vi "grain bin indicator debug.vi"() -> ()   [LabVIEW 2020]
panel:
  out "Numeric 2":dbl caption="bu"
  out "Numeric":dbl caption="bu"
  out "Boolean":bool
  out "Boolean 2":bool
  out "Boolean 4":bool
  out "Boolean 3":bool
  out "Slide 3":cluster{u8, u8}(slide)={0, 61}
  # "Dry Bin Storage"
  # "Dryer Bin"
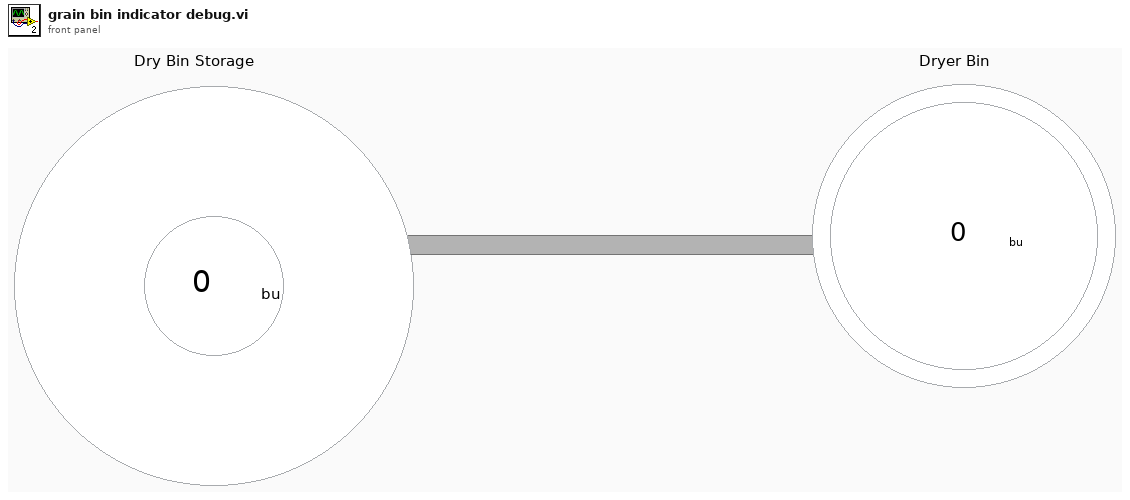
[diagram p1: front panel]
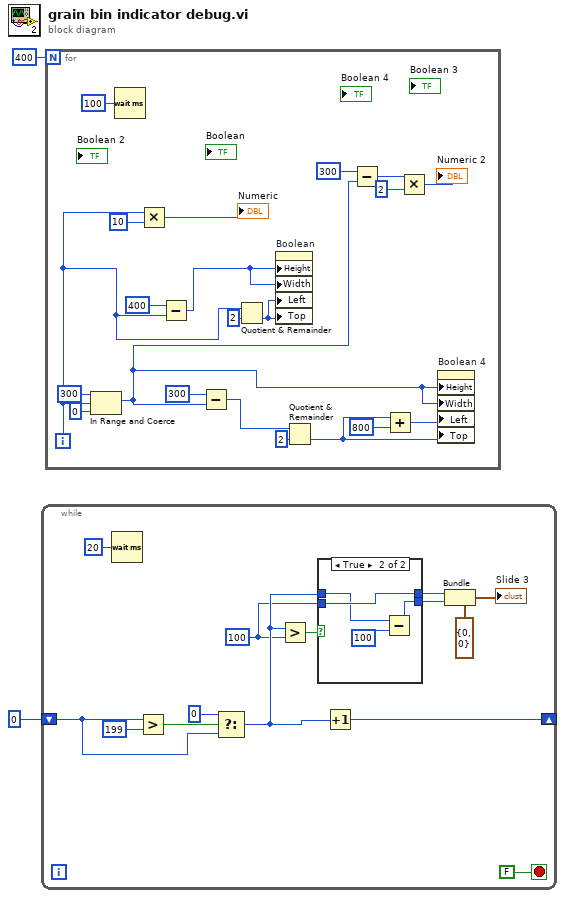
[diagram p0: block diagram]
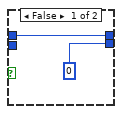
[diagram p2: hidden frame]
diagram:
  n1 = while {
    shift-right: [w14] -> _
    shift-left: u8 0 ("Slide") -> [w11]
    stop <- FALSE stop-if-true
    w4 = u8 100 ("y")
    n2 = Wait (ms)(milliseconds to wait=u32 20) -> ()  [unwired: 1 out]
    n3 = Greater?(x=w11, y=u8 199) -> (0:w12:bool)
    n4 = Select(t=u8 0, s=w12, f=w11) -> (s? t:f=w6:u8)
    n5 = Greater?(x=w6, y=w4) -> (0:w7:bool)
    n6 = case shown="True" w7 {
      tunnel: [w18 w22] -> w5
      tunnel: w6 -> [w18 w20]
      tunnel: w4 -> [_ w22]
      tunnel: [u8 0 ("t") w21] -> w3
      frame False {
      }
      frame True {
        n7 = Subtract(x=w20, y=u8 100) -> (x-y=w21:u8)
      }
    }
    n8 = Increment(x=w6) -> (x+1=w14:u8)
    n9 = Bundle(cluster=cluster{u8, u8} {0, 0} ("Slide 2"), w5, w3) -> (→"Slide 3":cluster{u8, u8})
  }
  n10 = for {
    N: 400 -> [_]
    i -> [w27]
    n11 = In Range and Coerce(upper limit=300, x=w27, lower limit=0) -> (coerced(x)=w23:i32)  [unwired: 1 out]
    n12 = Wait (ms)(milliseconds to wait=u32 100) -> ()  [unwired: 1 out]
    n13 = Multiply(x=w27, y=10) -> (x*y=→"Numeric":i32)
    n14 = Subtract(x=400, y=w27) -> (x-y=w39:i32)
    n15 = Subtract(x=300, y=w23) -> (x-y=w32:i32)
    n16 = Quotient & Remainder(x=w27, y=2) -> (floor(x/y)=w40:i32)  [unwired: 1 out]
    n17 = property on="Boolean" class="Bool (strict)"("Height"=w39, "Width"=w39, "Left"=w40, "Top"=w40) -> ()  [unwired: 2 in, 2 out]
    n18 = Quotient & Remainder(x=w32, y=2) -> (floor(x/y)=w33:i32)  [unwired: 1 out]
    n19 = Subtract(x=300, y=w23) -> (x-y=w25:i32)
    n20 = Add(x=w33, y=800) -> (x+y=w34:i32)
    n21 = Multiply(x=w25, y=2) -> (x*y=→"Numeric 2":i32)
    n22 = property on="Boolean 4" class="Bool (strict)"("Height"=w23, "Width"=w23, "Left"=w34, "Top"=w33) -> ()  [unwired: 2 in, 2 out]
  }
